vi "convertToSalStart.vi"(8 "error in (no error)":errorcluster, 10 "Configuration":string, 11 "CommandConstruction in":refnum<class "CommandConstruction.lvclass">) -> (0 "error out":errorcluster, 3 "CommandConstruction out":refnum<class "CommandConstruction.lvclass">)   [LabVIEW 2016, in "StartSAL.lvclass"]
uses:
  StartSAL.lvclass
  CommandConstruction/CommandConstruction.lvclass
  home/andres/ct_cmpuserevents/ComponentTemplateCore/ComponentModel/ComponentModel/Command/Command.lvclass
  CommandConstruction/CommandConstruction.lvclass/CommandConstruction.ctl
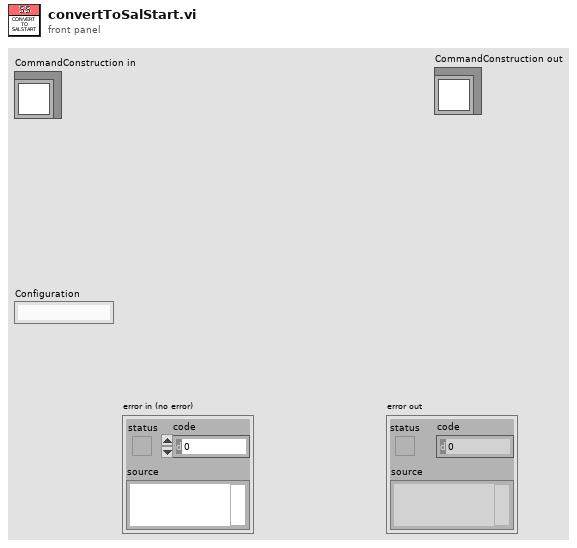
[diagram p1: front panel]
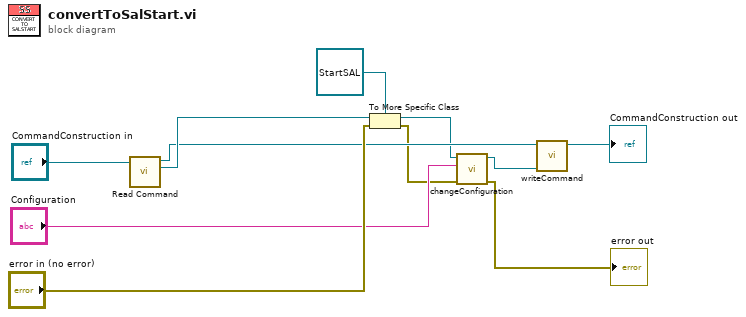
[diagram p0: block diagram]
diagram:
  n1 = call "Read Command.vi"("CommandConstruction in"="CommandConstruction in") -> ("Command.lvclass"=w10:refnum<class "Command.lvclass">, "CommandConstruction out"=w7:refnum<class "CommandConstruction.lvclass">)  [unwired: 9 in]
  n2 = To More Specific Class(target class=refnum<class "StartSAL.lvclass"> refnum ("StartSAL.lvclass"), reference=w10, error in="error in (no error)") -> (specific class reference=w1:refnum<class "StartSAL.lvclass">, error out=w4:errorcluster)
  n3 = call "changeConfiguration.vi"("error in (no error)"=w4, "configuration"="Configuration", "StartSAL.lvclass in"=w1) -> ("error out"=→"error out":errorcluster, "StartSAL.lvclass out"=w2:refnum<class "StartSAL.lvclass">)  [unwired: 7 in]
  n4 = call "writeCommand.vi"("Command.lvclass"=w2, "CommandConstruction in"=w7) -> ("CommandConstruction out"=→"CommandConstruction out":refnum<class "CommandConstruction.lvclass">)  [unwired: 9 in]
